vi "CANOpen_Get Section References by GUID.vi"(8 "error in (no error)":errorcluster, 10 "Search GUID":string="d746360c-3e97-4e77-b411-872b8f57c1d4", 11 "Device Ref":T1 format="%.0x") -> (0 "error out":errorcluster, 2 "Data References":T2 {"Hardware Output"."Channel Pairs"."Chan Refs" format="%.0x"}, 3 "Device Ref out":T1=18446744073709551615 format="%.0x")   [LabVIEW 2011]
uses:
  <vilib>/NI Veristand/Custom Device API/Custom Device Item Ref.ctl
  CANOpen_VS Bidirectional Data Refs.ctl
  <vilib>/NI Veristand/Custom Device API/Data Reference.ctl
  <vilib>/NI Veristand/Custom Device Tools/Custom Device Utility Library/NI VeriStand - Search for Item by GUID.vi
  <vilib>/NI Veristand/Custom Device API/NI VeriStand - Get Channel Data Reference.vi
  <vilib>/NI Veristand/Custom Device API/Custom Device API.lvlib
  <vilib>/NI Veristand/Custom Device Tools/Custom Device Utility Library/Custom Device Utility Library.lvlib
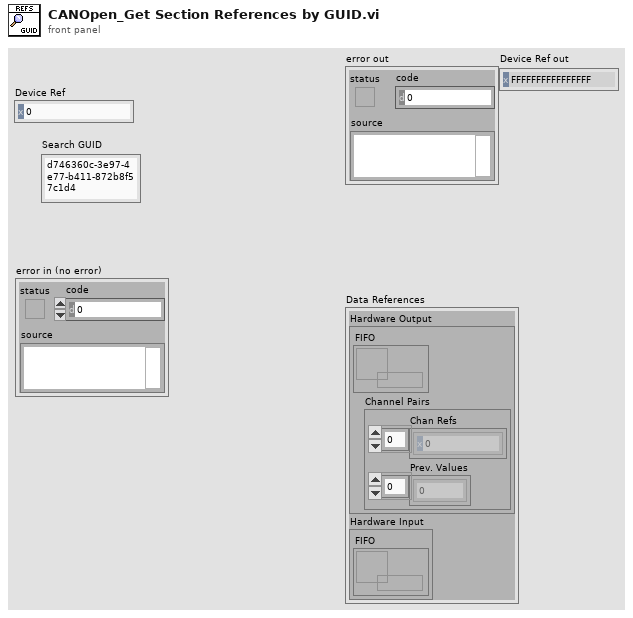
[diagram p1: front panel]
types:
  T1 = typedef "Custom Device API.lvlib/Custom Device Item Ref.ctl" = u64
  T2 = typedef "CANOpen_VS Bidirectional Data Refs.ctl" = cluster{"Hardware Output":cluster{"FIFO":refnum<k33>, "Channel Pairs":cluster{"Chan Refs":T3[], "Prev. Values":dbl[]}}, "Hardware Input":cluster{"FIFO":refnum<k33>}}
  T3 = typedef "Custom Device API.lvlib/Data Reference.ctl" = i32
  T4 = typedef "Custom Device API.lvlib/Custom Device Item Info.ctl" = cluster{"Name":string, "Is Channel":bool, "GUID":string}
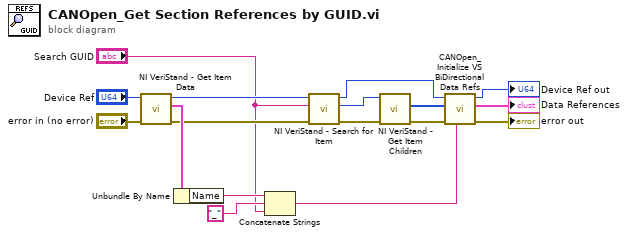
[diagram p0: block diagram]
diagram:
  n1 = call <vilib>:"NI VeriStand - Get Item Data.vi"("error in (no error)"="error in (no error)", "Item Ref in"="Device Ref") -> ("error out"=w10:errorcluster, "Item Info"=w17:T4, "Item Ref out"=w9:T1)  [unwired: 6 in, 1 out]
  n2 = Unbundle By Name(w17) -> ("Name"=w14:string)
  n3 = Concatenate Strings(w14, "_" ("string"), "Search GUID") -> (w8:string)
  n4 = call-poly <vilib>:"NI VeriStand - Search for Item.vi"("error in"=w10, "Item GUID"="Search GUID", "Section Ref in"=w9) -> ("error out"=w12:errorcluster, "Item Ref"=w11:T1, "Section Ref out"=w7:T1)  [unwired: 5 in, 1 out]
  n5 = call <vilib>:"NI VeriStand - Get Item Children.vi"("error in (no error)"=w12, "Item Ref in"=w11) -> ("error out"=w6:errorcluster, "Child Refs"=w1:T1[])  [unwired: 6 in, 2 out]
  n6 = call "CANOpen_Initialize VS BiDirectional Data Refs.vi"("Name"=w8, "error in (no error)"=w6, "Hardware Output Refs"=w1, "Device Ref"=w7) -> ("error out"=→"error out":errorcluster, "Data References"=→"Data References":T2, "Device Ref out"=→"Device Ref out":T1)  [unwired: 5 in]
